vi "Array of VData to VCluster__ogtk.vi"(8 "error in (no error)":errorcluster, 9 "Cluster Name":string, 10 "Array":variant[](array[variant])) -> (0 "error out":errorcluster, 2 "VCluster":variant)   [LabVIEW 2018]
doc: "Returns the elements of an array as elements of a variant cluster."
uses:
  <userlib>/_OpenG.lib/lvdata/lvdata.llb/Type Descriptor Enumeration__ogtk.ctl
panel:
  # "[OpenG VI Tags] ***Do Not Remove***"
  # "Array of VData to VCluster.vi\n\nReturns the elements of an array as elements of a variant cluster.\n\nPlease visit http://www.OpenG.org to learn about the\nOpen Source LabVIEW software movement.\n\nNOTICE -- YOU MUST LEAVE THIS NOTICE IN PLACE.  PER THE TERMS OF THE LICENSE BELOW, YOU MAY SUBLICENSE THIS SOFTWARE \nIN ANY WAY THAT DOES NOT CONFLICT WITH THIS LICENSE.\n\n### BSD License (http://www.opensource.org/licenses/bsd-license.php) Begin ###\n \nCopyright (c) 2002, Jean-Pierre Drolet <drolet_jp@hotmail.com>\nCopyright (c) 2002-2006, Jim Kring <jim@jimkring.com>\n\nAll rights reserved.\n\nRedistribution and use in source and binary forms, with or without modification, are permitted provided that the following conditions are met:\n\n    * Redistributions of source code must retain the above copyright notice, this list of conditions and the following disclaimer.\n    * Redistributions in binary form must reproduce the above copyright notice, this list of conditions and the following disclaimer in the \n       documentation and/or other materials provided with the distribution.\n    * Neither the name of SciWare, James Kring, Inc., nor the names of its contributors may be used to endorse or promote products derived \n       from this software without specific prior written permission.\n\nTHIS SOFTWARE IS PROVIDED BY THE COPYRIGHT HOLDERS AND CONTRIBUTORS \"AS IS\" AND ANY EXPRESS OR IMPLIED WARRANTIES, \nINCLUDING, BUT NOT LIMITED TO, THE IMPLIED WARRANTIES OF MERCHANTABILITY AND FITNESS FOR A PARTICULAR PURPOSE ARE \nDISCLAIMED. IN NO EVENT SHALL THE COPYRIGHT OWNER OR CONTRIBUTORS BE LIABLE FOR ANY DIRECT, INDIRECT, INCIDENTAL,\n SPECIAL, EXEMPLARY, OR CONSEQUENTIAL DAMAGES (INCLUDING, BUT NOT LIMITED TO, PROCUREMENT OF SUBSTITUTE GOODS OR \nSERVICES; LOSS OF USE, DATA, OR PROFITS; OR BUSINESS INTERRUPTION) HOWEVER CAUSED AND ON ANY THEORY OF LIABILITY, \nWHETHER IN CONTRACT, STRICT LIABILITY, OR TORT (INCLUDING NEGLIGENCE OR OTHERWISE) ARISING IN ANY WAY OUT OF THE USE \nOF THIS SOFTWARE, EVEN IF ADVISED OF THE POSSIBILITY OF SUCH DAMAGE.\n\n### BSD License End ###"
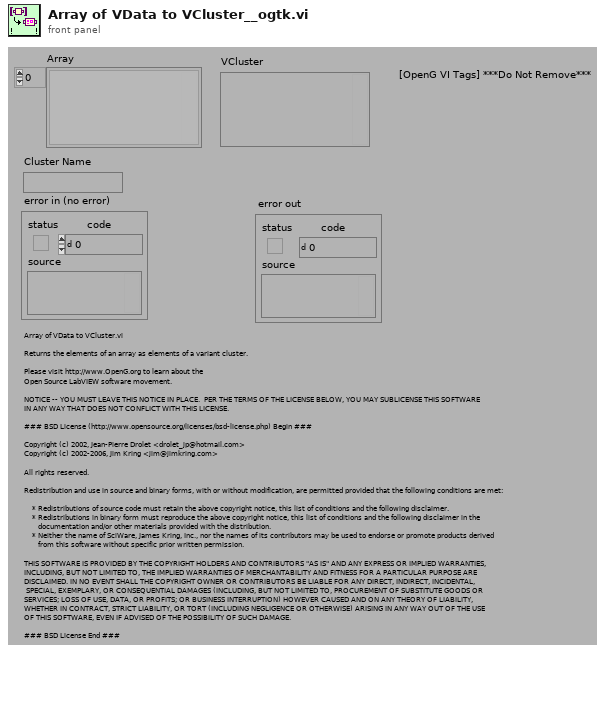
[diagram p1: front panel]
types:
  T1 = typedef "Type Descriptor Enumeration__ogtk.ctl" = enum8{"<Null>", "I8", "I16", "I32", "I64", "U8", "U16", "U32", "U64", "SGL", "DBL", "EXT", "CSG", "CDB", "CXT", "0x0F", "0x10", "0x11", "0x12", "0x13", "0x14", "Enum U8", "Enum U16", "Enum U32", "Enum U64", "SGL PQ", "DBL PQ", "EXT PQ", "CSG PQ", "CDB PQ", "CXT PQ", "0x1F", "0x20", "Boolean", "0x22", "0x23", "0x24", "0x25", "0x26", "0x27", "0x28", "0x29", "0x2A", "0x2B", "0x2C", "0x2D", "0x2E", "0x2F", "String", "0x31", "Path", "Pict", "0x34", "0x35", "0x36", "DAQ", "0x38", "0x39", "0x3A", "0x3B", "0x3C", "0x3D", "0x3E", "0x3F", "Array", "0x41", "0x42", "0x43", "0x44", "0x45", "0x46", "0x47", "0x48", "0x49", "0x4A", "0x4B", "0x4C", "0x4D", "0x4E", "0x4F", "Cluster", "0x51", "0x52", "Variant", "Waveform", "0x55", "0x56", "0x57", "0x58", "0x59", "0x5A", "0x5B", "0x5C", "0x5D", "0x5E", "0x5F", "0x60", "0x61", "0x62", "0x63", "0x64", "0x65", "0x66", "0x67", "0x68", "0x69", "0x6A", "0x6B", "0x6C", "0x6D", "0x6E", "0x6F", "Refnum"}
  T2 = typedef "Type Descriptor__ogtk.ctl" = i16[]
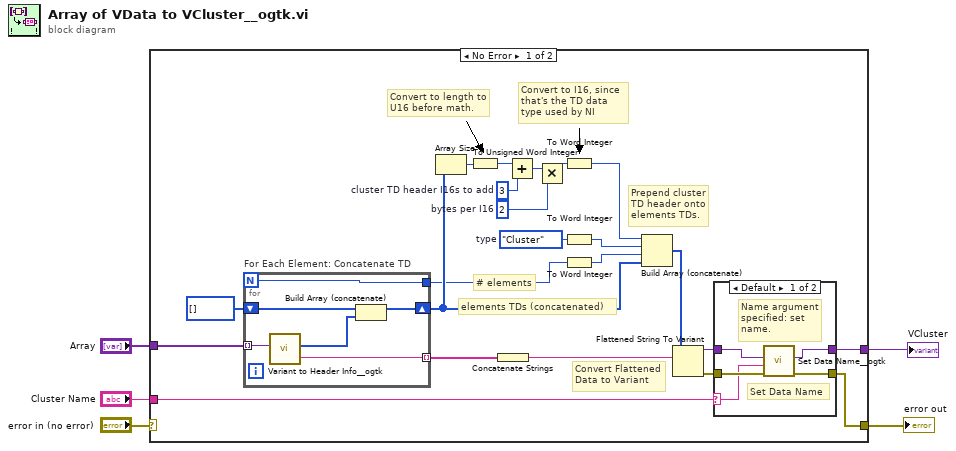
[diagram p0: block diagram]
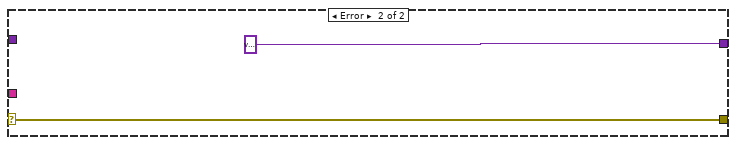
[diagram p3: hidden frame]
diagram:
  n1 = case shown="No Error" "error in (no error)" {
    selector: "error in (no error)" -> [_ w42]
    tunnel: [w14 w42] -> w5
    tunnel: [w16 variant ("Variant")] -> w3
    tunnel: "Array" -> [w18 _]
    tunnel: "Cluster Name" -> [w17 _]
    frame No Error {
      w8 = u16 2  # bytes per I16
      w10 = u16 3  # cluster TD header I16s to add
      w20 = Type_Descriptor_Enumeration__ogtk."Cluster"  # type
      # "Convert Flattened Data to Variant"
      # "elements TDs (concatenated)"
      # "Convert to length to U16 before math."
      # "Convert to I16, since that's the TD data type used by NI"
      # "Prepend cluster TD header onto elements TDs."
      # "# elements"
      n2 = for "For Each Element: Concatenate TD" {
        N -> [w35]
        tunnel: w18 -> [w40] mode=indexing
        tunnel: [w39] -> w27 mode=indexing
        shift-right: [w37] -> w21
        shift-left: i16[] [] -> [w36]
        tunnel: [w35] -> w11
        n3 = call <userlib>:"Variant to Header Info__ogtk.vi"("Variant"=w40) -> ("Type Descriptor"=w38:T2, "data string"=w39:string)  [unwired: 3 in, 1 out]
        n4 = Build Array (concatenate)(w36, w38) -> (w37:T2)
      }
      n5 = Array Size(array=w21) -> (size(s)=w23:i32)
      n6 = To Unsigned Word Integer(number=w23) -> (unsigned 16bit integer=w7:u16)
      n7 = Concatenate Strings(w27) -> (w25:string)
      n8 = Add(x=w7, y=w10) -> (x+y=w9:u16)
      n9 = Multiply(x=w9, y=w8) -> (x*y=w6:u16)
      n10 = To Word Integer(number=w6) -> (16bit integer=w22:i16)
      n11 = To Word Integer(number=w20) -> (16bit integer=w12:i16)
      n12 = To Word Integer(number=w11) -> (16bit integer=w19:i16)
      n13 = Build Array (concatenate)(w22, w12, w19, w21) -> (w24:T2)
      n14 = Flattened String To Variant(6:w25, 7:w24) -> (0:w13:errorcluster, 3:w15:variant)  [unwired: 1 in]
      n15 = case shown="Default" w17 {
        selector: w17 -> [w30 _]
        tunnel: [w28 w34] -> w16
        tunnel: w15 -> [w29 w34]
        tunnel: [w31 w33] -> w14
        tunnel: w13 -> [w32 w33]
        frame Default {
          # "Set Data Name"
          # "Name argument specified: set name."
          n16 = call <userlib>:"Set Data Name__ogtk.vi"("error in (no error)"=w32, "Data Name"=w30, "Data"=w29) -> ("error out"=w31:errorcluster, "Renamed Data"=w28:variant)  [unwired: 7 in]
        }
        frame "" {
          # "Name argument is empty: don't set name."
        }
      }
    }
    frame Error {
    }
  }
  "error out" <- w5
  "VCluster" <- w3
